vi "Create Voltage Input.vi"(8 "error in (no error)":errorcluster, 10 "Params":variant, 11 "NI Analog Input in":refnum<class "NI Analog Input.lvclass">) -> (0 "error out":errorcluster, 3 "NI Analog Input out":refnum<class "NI Analog Input.lvclass">)   [LabVIEW 2020, in "NI DAQmx.lvlib" / "NI Analog Input.lvclass"]
uses:
  NI Analog Input.lvclass
  D:/WSGitHub/RTFWK/Realization/NI DAQmx Base/NI DAQmx Base.lvclass
  NI DAQmx Base/TypeDefs/Channel Config.ctl
  <vilib>/DAQmx/create/channels.llb/DAQmx Create Channel (AI-Voltage-Basic).vi
  NI Analog Input.lvclass/NI Analog Input.ctl
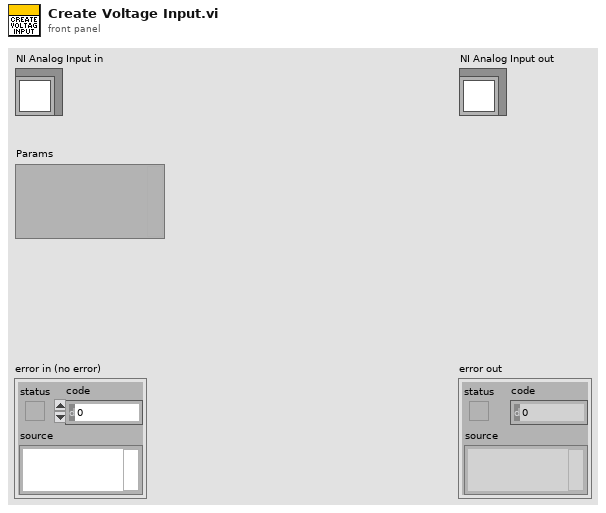
[diagram p1: front panel]
types:
  T1 = typedef "Channel Config.ctl" = cluster{"channels":string, "maximum value":dbl, "minimum value":dbl, "output terminal configuration":i32, "units":i32}
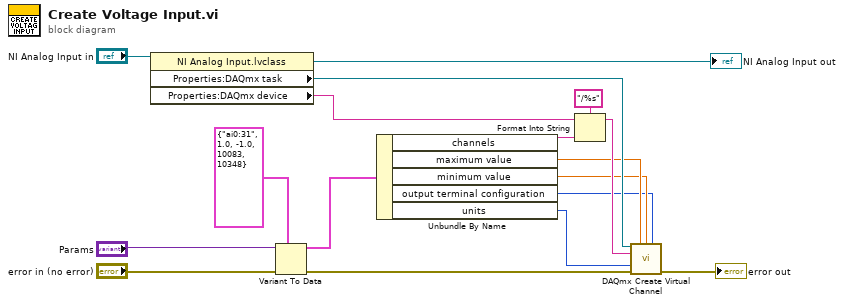
[diagram p0: block diagram]
diagram:
  n1 = property class="NI Analog Input.lvclass"(reference="NI Analog Input in") -> (reference out=→"NI Analog Input out":refnum<class "NI Analog Input.lvclass">, "Properties:DAQmx task"=w15:refnum<k21>, "Properties:DAQmx device"=w16:tag)  [unwired: 1 in, 1 out]
  n2 = Variant To Data(error in="error in (no error)", type=T1 {"channels"="ai0:31", "maximum value"=1.0, "minimum value"=-1.0, "output terminal configuration"=10083, "units"=10348} ("Channel Config"), Variant="Params") -> (data=w7:T1, error out=w17:errorcluster)
  n3 = Unbundle By Name(w7) -> ("channels"=w13:string, "maximum value"=w11:dbl, "minimum value"=w10:dbl, "output terminal configuration"=w9:i32, "units"=w8:i32)
  n4 = Format Into String(format string="/%s", initial string=w16, w13) -> (resulting string=w12:string)  [unwired: 1 in, 1 out]
  n5 = call-poly <vilib>:"DAQmx Create Virtual Channel.vi"("task in"=w15, "maximum value"=w11, "minimum value"=w10, "input terminal configuration"=w9, "physical channels"=w12, "units"=w8, "error in"=w17) -> ("error out"=→"error out":errorcluster)  [unwired: 7 in, 1 out]
